vi "citTemplate.queueRepository.vi"(0 "mode (get queue handle)":T3=enum."get queue handle(s)", 1 "queue in":refnum<queue>, 2 "instance (0)":i32, 7 "event in":variant, 9 "(flatten) data in":string, 11 "error in (no error)":errorcluster) -> (3 "queue out":refnum<queue>, 4 "queueHandle(s) out":refnum<queue>[](array[refnum]), 8 "eventIndex(s)":u32[](array[numeric]), 15 "error out":errorcluster)   [LabVIEW 2019, in "Tools.lvlib"]
uses:
  Tools.lvlib
  citTemplate.eventQueue.ctl
  citTemplate.queueData.ctl
  citTemplate.notifierHandle.ctl
  citTemplate.notifierData.ctl
  citTemplate.ackNotifier.ctl
  citTemplate.ackData.ctl
panel:
  in  "queueData":T1
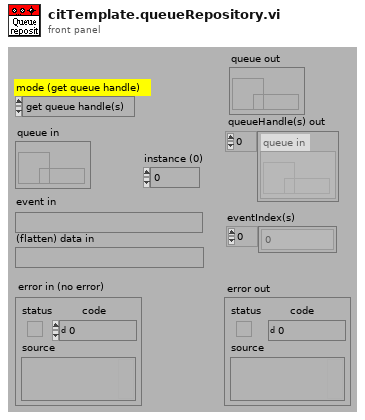
[diagram p1: front panel]
types:
  T1 = typedef "Tools.lvlib/citTemplate.queueData.ctl" = cluster{"event index":u32, "(flatten) data in":string, "notifierHandle":T2}
  T2 = typedef "Tools.lvlib/citTemplate.notifierHandle.ctl" = refnum<notifier>
  T3 = typedef "Tools.lvlib/citTemplate.eventQueue.ctl" = enum16{"create queue", "get queue handle(s)", "destroy queue"}
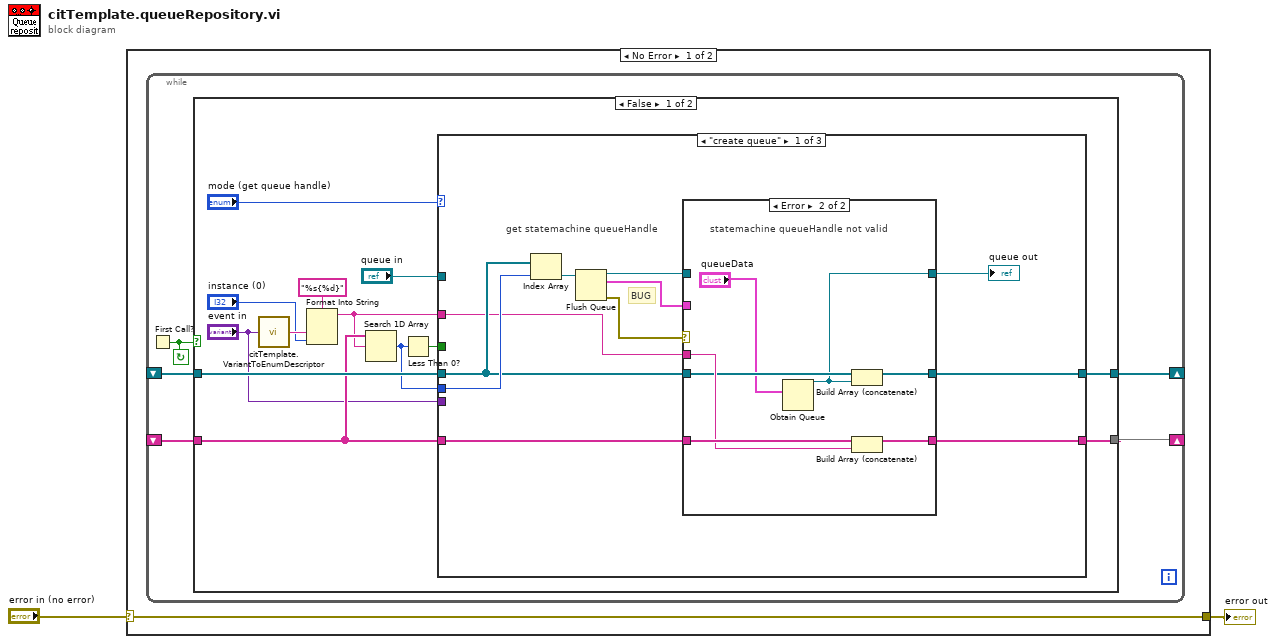
[diagram p0: block diagram]
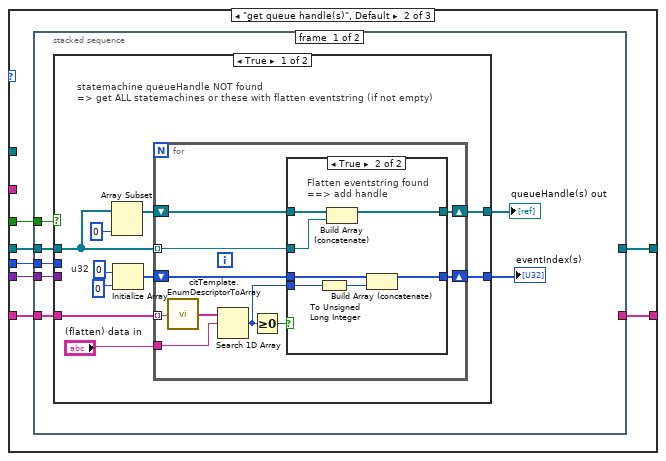
[diagram p3: hidden frame]
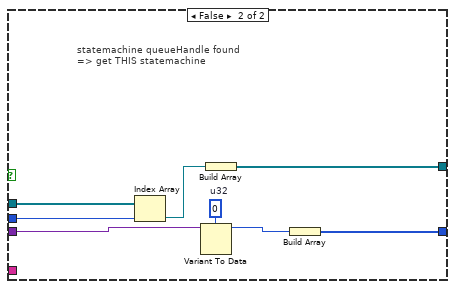
[diagram p5: hidden frame]
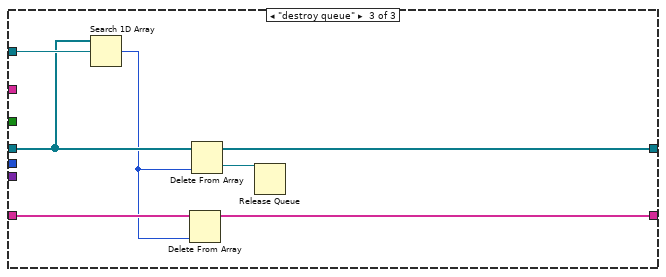
[diagram p7: hidden frame]
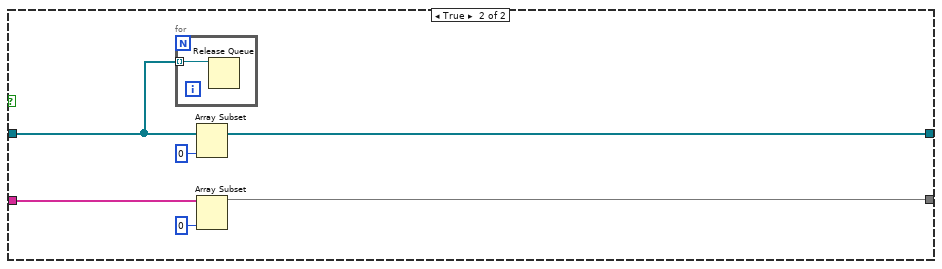
[diagram p8: hidden frame]
diagram:
  n1 = case shown="No Error" "error in (no error)" {
    selector: "error in (no error)" -> [w3 w110]
    tunnel: [w3 w110] -> w1
    frame No Error {
      n2 = while {
        shift-right: [w8] -> _
        shift-left: _ -> [w5]
        shift-right: [w7] -> _
        shift-left: _ -> [w6]
        stop <- w4 continue-if-true
        n3 = First Call?() -> (First Call?: T/F=w4:bool)
        n4 = case shown="False" w4 {
          tunnel: [w21 w104] -> w8
          tunnel: [w20 w105] -> w7
          tunnel: w6 -> [w19 w103]
          tunnel: w5 -> [w15 w106]
          frame False {
            n5 = call "citTemplate.VariantToEnumDescriptor.vi"("Variant enum data"="event in") -> ("enum type descriptor"=w12:string)  [unwired: 14 out]
            n6 = Format Into String(format string="%s{%d}", w12, "instance (0)") -> (resulting string=w10:string)  [unwired: 2 in, 1 out]
            n7 = Search 1D Array(1D array=w15, element=w10) -> (index of element=w16:i32)  [unwired: 1 out]
            n8 = Less Than 0?(x=w16) -> (x < 0?=w17:bool)
            n9 = case shown="\"create queue\"" "mode (get queue handle)" {
              tunnel: [w26 w49 w98] -> w21
              tunnel: [w28 w48 w97] -> w20
              tunnel: w19 -> [w29 w47 w101]
              tunnel: w15 -> [w27 w46 w100]
              tunnel: w10 -> [w23 _ _]
              tunnel: w17 -> [_ w44 _]
              tunnel: w16 -> [w32 w45 _]
              tunnel: "queue in" -> [_ _ w102]
              tunnel: "event in" -> [_ w43 _]
              frame "create queue" {
                # "BUG"
                # "get statemachine queueHandle"
                n10 = Index Array(array=w29, index=w32) -> (element=w31:refnum<queue>)
                n11 = Flush Queue(queue=w31) -> (queue out=w30:refnum<queue>, remaining elements=w24:T1[], error out=w25:errorcluster)  [unwired: 1 in]
                n12 = case shown="Error" w25 {
                  tunnel: w27 -> [w35 w42]
                  tunnel: w23 -> [_ w41]
                  tunnel: w29 -> [w34 w40]
                  tunnel: [w34 w39] -> w28
                  tunnel: [w35 w38] -> w26
                  tunnel: [w33 w37] -> w22
                  tunnel: w30 -> [w33 _]
                  tunnel: w24 -> [_ _]
                  frame No Error {
                    # "statemachine queueHandle valid"
                  }
                  frame Error {
                    # "statemachine queueHandle not valid"
                    n13 = Obtain Queue(element data type="queueData") -> (queue out=w37:refnum<queue>)  [unwired: 3 in, 3 out]
                    n14 = Build Array (concatenate)(w40, w37) -> (w39:refnum<queue>[])
                    n15 = Build Array (concatenate)(w42, w41) -> (w38:string[])
                  }
                }
                "queue out" <- w22
              }
              frame "get queue handle(s)", Default {
                n16 = stacked-sequence {
                  tunnel: w46 -> [w53 w94]
                  tunnel: [_ w95] -> w48
                  tunnel: w47 -> [w56 w95]
                  tunnel: [_ w94] -> w49
                  tunnel: w45 -> [w55 _]
                  tunnel: w44 -> [w54 _]
                  tunnel: w43 -> [w50 _]
                  frame #0 {
                    n17 = case shown="True" w54 {
                      tunnel: w56 -> [w65 w93]
                      tunnel: w55 -> [_ w91]
                      tunnel: w53 -> [w66 _]
                      tunnel: [w58 w89] -> w52
                      tunnel: [w57 w90] -> w51
                      tunnel: w50 -> [_ w86]
                      frame True {
                        w60 = u32 0  # u32
                        # "statemachine queueHandle NOT found\n=> get ALL statemachines or these with flatten eventstring (if not empty)"
                        n18 = Array Subset(array=w65, length=0) -> (w63:refnum<queue>[])  [unwired: 1 in]
                        n19 = Initialize Array(w60, 0 ("length")) -> (w61:u32[])
                        n20 = for {
                          tunnel: w65 -> [w76] mode=indexing
                          tunnel: w66 -> [w75] mode=indexing
                          tunnel: "(flatten) data in" -> [w73]
                          shift-right: [w70] -> w58
                          shift-left: w63 -> [w71]
                          shift-right: [w67] -> w57
                          shift-left: w61 -> [w69]
                          n21 = call "citTemplate.EnumDescriptorToArray.vi"("enum type descriptor"=w75) -> ("array"=w74:string[])  [unwired: 14 out]
                          n22 = Search 1D Array(1D array=w74, element=w73) -> (index of element=w68:i32)  [unwired: 1 out]
                          n23 = Greater Or Equal To 0?(x=w68) -> (x >= 0?=w72:bool)
                          n24 = case shown="True" w72 {
                            tunnel: w76 -> [_ w84]
                            tunnel: w71 -> [w78 w85]
                            tunnel: [w78 w83] -> w70
                            tunnel: w69 -> [w77 w80]
                            tunnel: w68 -> [_ w82]
                            tunnel: [w77 w79] -> w67
                            frame False {
                              # "Flatten eventstring not found"
                            }
                            frame True {
                              # "Flatten eventstring found\n==> add handle"
                              n25 = To Unsigned Long Integer(number=w82) -> (unsigned 32bit integer=w81:u32)
                              n26 = Build Array (concatenate)(w85, w84) -> (w83:refnum<queue>[])
                              n27 = Build Array (concatenate)(w80, w81) -> (w79:u32[])
                            }
                          }
                        }
                      }
                      frame False {
                        w88 = u32 0  # u32
                        # "statemachine queueHandle found\n=> get THIS statemachine"
                        n28 = Index Array(array=w93, index=w91) -> (element=w92:refnum<queue>)
                        n29 = Variant To Data(type=w88, Variant=w86) -> (data=w87:u32)  [unwired: 1 in, 1 out]
                        n30 = Build Array(w92) -> (w89:refnum<queue>[])
                        n31 = Build Array(w87) -> (w90:u32[])
                      }
                    }
                    "queueHandle(s) out" <- w52
                    "eventIndex(s)" <- w51
                  }
                  frame #1 {
                    # "datatunnel"
                  }
                }
              }
              frame "destroy queue" {
                n32 = Search 1D Array(1D array=w101, element=w102) -> (index of element=w99:i32)  [unwired: 1 out]
                n33 = Delete From Array(array=w100, index=w99) -> (array with subset deleted=w98:string[])  [unwired: 1 in, 1 out]
                n34 = Delete From Array(array=w101, index=w99) -> (deleted portion=w96:refnum<queue>, array with subset deleted=w97:refnum<queue>[])  [unwired: 1 in]
                n35 = Release Queue(queue=w96) -> ()  [unwired: 1 in, 4 out]
              }
            }
          }
          frame True {
            n36 = for {
              tunnel: w103 -> [w109] mode=indexing
              n37 = Release Queue(queue=w109) -> ()  [unwired: 1 in, 4 out]
            }
            n38 = Array Subset(array=w103, length=0) -> (w105:refnum<queue>[])  [unwired: 1 in]
            n39 = Array Subset(array=w106, length=0) -> (w104:string[])  [unwired: 1 in]
          }
        }
      }
    }
    frame Error {
    }
  }
  "error out" <- w1
